vi "Traffic Light Main.vi"() -> ()   [LabVIEW 2020]
uses:
  Traffic.ctl
panel:
  in  "stop":bool
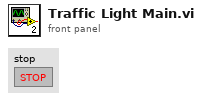
[diagram p1: front panel]
types:
  T1 = typedef "Traffic.ctl" = enum16{"H-Go", "H-Warning", "H-Finishing", "H-Stop", "V-Go", "V-Warning", "V-Finishing", "V-Stop"}
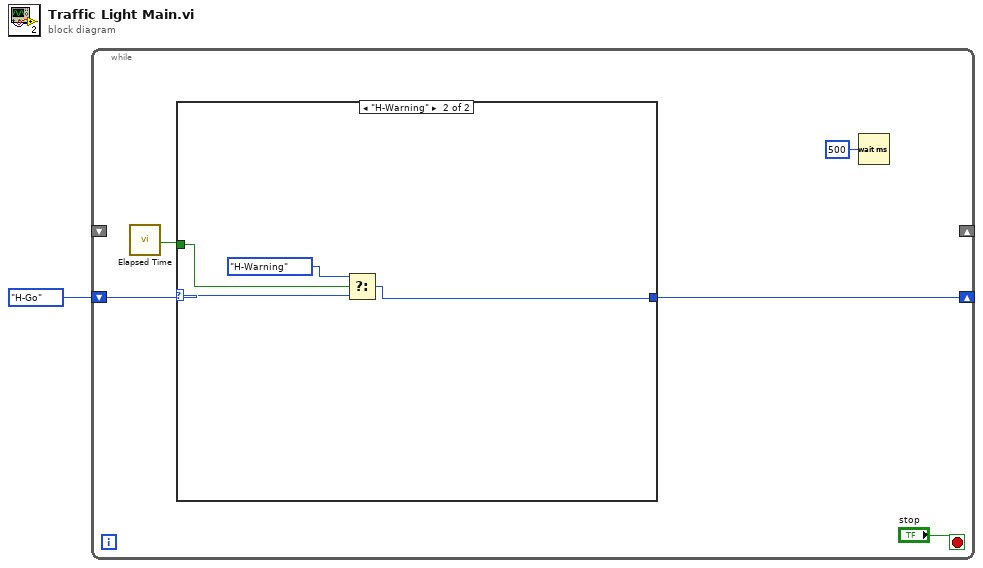
[diagram p0: block diagram]
diagram:
  n1 = while {
    shift-right: [w4] -> _
    shift-left: Traffic."H-Go" -> [w6]
    shift-right: _ -> [_]
    shift-left: _ -> [_]
    stop <- "stop" stop-if-true
    n2 = call "Elapsed Time"() -> ("Time has Elapsed"=w5:bool)  [unwired: 12 in, 7 out]
    n3 = case shown="\"H-Warning\"" w6 {
      selector: w6 -> [_ w10]
      tunnel: w5 -> [_ w9]
      tunnel: [_ w7] -> w4
      frame "H-Go", Default {
      }
      frame "H-Warning" {
        n4 = Select(t=Traffic."H-Warning", s=w9, f=w10) -> (s? t:f=w7:T1)
      }
    }
    n5 = Wait (ms)(milliseconds to wait=u32 500 ("millisecond timer value")) -> ()  [unwired: 1 out]
  }
